vi "WAI.vi"(0 "System no.":i32=1 min=1 max=4 step=1, 2 "Affected axes?":string[](array[string]), 3 "All axes?":bool, 4 "Axis identifier?":bool=TRUE, 5 "error in":errorcluster) -> (19 "error out":errorcluster)   [LabVIEW 2020]
doc: "This VI sends the wait command WAI to the controller. Controller will wait for specified axes to stop before executing any other command. Since the controller does not indicate when the wait phase has finished, WAI.vi does not provide that information.\n\nC-702: If All axes = TRUE, then Axis identifier must be TRUE\nC-848: If All axes = TRUE, then Axis identifier must be TRUE\nC-880: If All axes = TRUE, then Axis identifier must be TRUE"
panel:
  # "This vi sends the wait command WAI to the controller.\nController will wait for specified axes to stop before executing\nany other command. Since the controller does not indicate when\nthe wait phase has finished, WAI.vi does not provide that information."
  # "If all axes: use"
  # "Wait for"
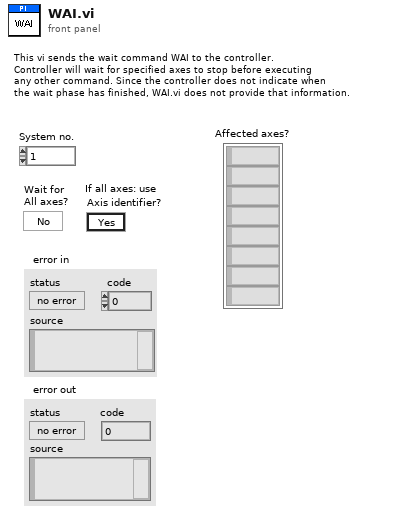
[diagram p1: front panel]
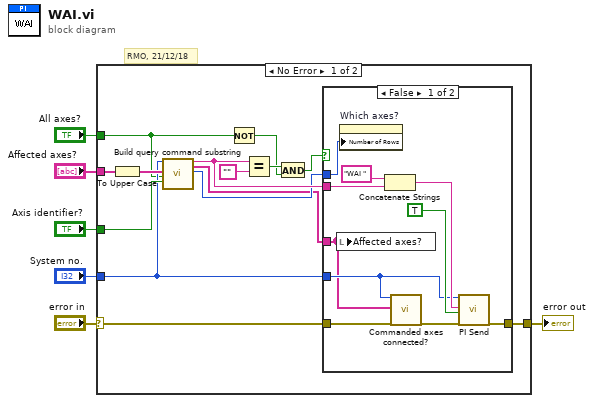
[diagram p0: block diagram]
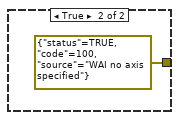
[diagram p2: hidden frame]
diagram:
  # "RMO, 21/12/18"
  n1 = case shown="No Error" "error in" {
    selector: "error in" -> [w9 w32]
    tunnel: "Affected axes?" -> [w20 _]
    tunnel: [w8 w32] -> w5
    tunnel: "Axis identifier?" -> [w17 _]
    tunnel: "System no." -> [w14 _]
    tunnel: "All axes?" -> [w12 _]
    frame No Error {
      n2 = To Upper Case(1:w20) -> (0:w18:string[])
      n3 = call "Build query command substring.vi"("System no."=w14, "Axes to query in"=w18, "Query\nAll axes?"=w12, "For all axes: use\nAxis identifier?"=w17) -> ("Command substring"=w16:string, "Axes to query out"=w13:string[], "Number of rows"=w15:u32)  [unwired: 2 in, 11 out]
      n4 = Not(x=w12) -> (.not. x?=w10:bool)
      n5 = Equal?(x=w16, y="" ("x")) -> (x = y?=w11:bool)
      n6 = And(x=w11, y=w10) -> (x .and. y?=w7:bool)
      n7 = case shown="False" w7 {
        tunnel: w16 -> [w27 _]
        tunnel: w15 -> [w26 _]
        tunnel: w14 -> [w25 _]
        tunnel: w13 -> [w24 _]
        tunnel: w9 -> [w22 _]
        tunnel: [w21 errorcluster {"status"=TRUE, "code"=100, "source"="WAI no axis specified"} ("error out")] -> w8
        frame False {
          n8 = local write "Affected axes?"(w24) -> ()
          n9 = property on="Which axes?" class="Arr (strict)"("Number of Rows"=w26) -> ()  [unwired: 2 in, 2 out]
          n10 = Concatenate Strings("WAI ", w27) -> (w28:string)
          n11 = call "Commanded axes connected?.vi"("System no."=w25, "Commanded axes"=w24, "error in"=w22) -> ("error out"=w23:errorcluster)  [unwired: 1 in, 15 out]
          n12 = call "PI Send.vi"("System no."=w25, "String to send"=w28, "Attach termination char.?"=TRUE ("Attach Linefeed?"), "error in"=w23) -> ("error out"=w21:errorcluster)  [unwired: 2 in, 13 out]
        }
        frame True {
        }
      }
    }
    frame Error {
    }
  }
  "error out" <- w5
